vi "UART Configuration Core.vi"(0 "FPGA VI Reference":T2, 1 "Channel Number":u8, 5 "Input Commands":T1[](array[typedef]), 7 "Input Parameters":u32[](array[numeric]), 11 "error in":errorcluster) -> (15 "error out":errorcluster)   [LabVIEW 2012, in "UART_Host_Driver.lvlib" / "UART Driver.lvclass"]
uses:
  UART Driver.lvclass
  Typedefs/FPGA VI Reference.ctl
  UART_Host_Driver.lvlib
  <vilib>/rvi/interface/nirviMethod/nirviMethod.xnode
  <vilib>/FPGAPlugInAG/Dynamic/niLvFpga_WriteFifo_Dynamic.vi
  <vilib>/rvi/errors/niLvFpgaMergeErrorWithErrorCode.vi
  FPGA/UART/UART_Command.ctl
  FPGA/UART/UART_Firmware.lvlib
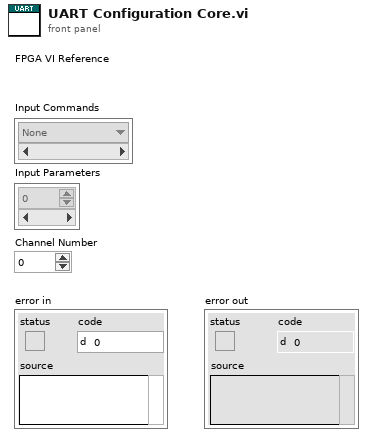
[diagram p1: front panel]
types:
  T1 = typedef "UART_Firmware.lvlib/UART_Command.ctl" = enum8{"None", "Tx", "SetBaud_High", "SetBaud_Low", "SetCharLength", "SetParity", "SetStopBits", "SetSpacing_High", "SetSpacing_Low"}
  T2 = typedef "UART_Host_Driver.lvlib/FPGA VI Reference.ctl" = refnum<k20>
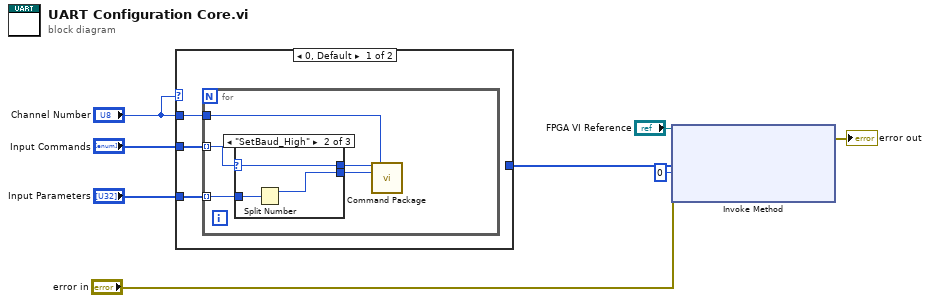
[diagram p0: block diagram]
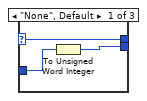
[diagram p2: hidden frame]
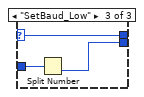
[diagram p3: hidden frame]
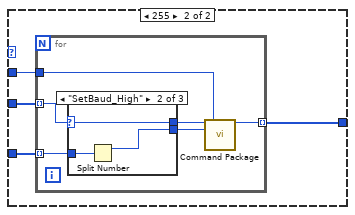
[diagram p4: hidden frame]
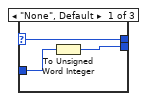
[diagram p5: hidden frame]
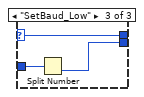
[diagram p6: hidden frame]
diagram:
  n1 = case shown="0, Default" "Channel Number" {
    tunnel: "Channel Number" -> [w11 w29]
    tunnel: [_ w28] -> w8
    tunnel: "Input Parameters" -> [w10 w27]
    tunnel: "Input Commands" -> [w9 w26]
    frame 0, Default {
      n2 = for {
        tunnel: w10 -> [w14] mode=indexing
        tunnel: w9 -> [w16] mode=indexing
        tunnel: w11 -> [w12]
        n3 = case shown="\"SetBaud_High\"" w16 {
          selector: w16 -> [w19 w22 w25]
          tunnel: [w19 w22 w25] -> w15
          tunnel: w14 -> [w18 w21 w24]
          tunnel: [w17 w20 w23] -> w13
          frame "None", Default {
            n4 = To Unsigned Word Integer(number=w18) -> (unsigned 16bit integer=w17:u16)
          }
          frame "SetBaud_High" {
            n5 = Split Number(x=w21) -> (hi(x)=w20:u16)  [unwired: 1 out]
          }
          frame "SetBaud_Low" {
            n6 = Split Number(x=w24) -> (lo(x)=w23:u16)  [unwired: 1 out]
          }
        }
        n7 = call "Command Package.vi"("UART_Command"=w15, "Channel Number"=w12, "Cmd_data"=w13) -> ()  [unwired: 12 in, 1 out]
      }
    }
    frame 255 {
      n8 = for {
        tunnel: [w33] -> w28 mode=indexing
        tunnel: w27 -> [w32] mode=indexing
        tunnel: w26 -> [w35] mode=indexing
        tunnel: w29 -> [w30]
        n9 = case shown="\"SetBaud_High\"" w35 {
          selector: w35 -> [w38 w41 w44]
          tunnel: [w38 w41 w44] -> w34
          tunnel: w32 -> [w37 w40 w43]
          tunnel: [w36 w39 w42] -> w31
          frame "None", Default {
            n10 = To Unsigned Word Integer(number=w37) -> (unsigned 16bit integer=w36:u16)
          }
          frame "SetBaud_High" {
            n11 = Split Number(x=w40) -> (hi(x)=w39:u16)  [unwired: 1 out]
          }
          frame "SetBaud_Low" {
            n12 = Split Number(x=w43) -> (lo(x)=w42:u16)  [unwired: 1 out]
          }
        }
        n13 = call "Command Package.vi"("UART_Command"=w34, "Channel Number"=w30, "Cmd_data"=w31) -> ("Cmd_package"=w33:u32)  [unwired: 12 in]
      }
    }
  }
  n14 = xnode "Invoke Method"("FPGA VI Reference In"="FPGA VI Reference", "error in"="error in", "Data"=w8, "Timeout (ms)"=0) -> ("error out"=→"error out":errorcluster)  [unwired: 2 out]
